vi "Newmark-Jog.vi"(0 "Table VRN IN":refnum<visa-resource-name>="COM9", 1 "StageTag":string, 2 "Bool Refnum":refnum<vi>, 11 "Error IN":errorcluster, 13 "Velocity":dbl) -> (4 "Table VRN OUT":refnum<visa-resource-name>="COM9", 15 "Error OUT":errorcluster)   [LabVIEW 2011]
uses:
  Comm/SerialCommError.vi
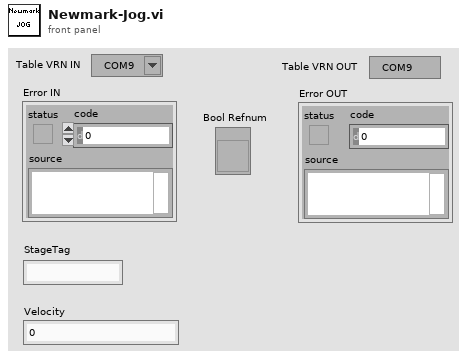
[diagram p1: front panel]
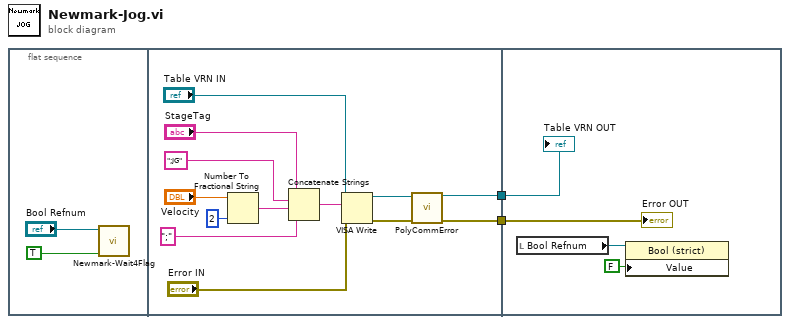
[diagram p0: block diagram]
diagram:
  n1 = flat-sequence {
    tunnel: [w15] -> w2
    tunnel: [w14] -> w1
    tunnel: w2 -> [w20]
    tunnel: w1 -> [w19]
    frame #0 {
      n2 = call "Newmark-Wait4Flag.vi"("Raise Flag ?"=TRUE, "Ctl Refnum IN"="Bool Refnum") -> ()  [unwired: 8 in, 2 out]
    }
    frame #1 {
      n3 = Number To Fractional String(number="Velocity", precision (6)=i16 2) -> (F-format string=w8:string)  [unwired: 2 in]
      n4 = Concatenate Strings("StageTag", ";JG", w8, ";") -> (w5:string)
      n5 = VISA Write(VISA resource name="Table VRN IN", write buffer=w5, error in (no error)="Error IN") -> (VISA resource name out=w17:refnum<visa-resource-name>, error out=w16:errorcluster)  [unwired: 1 out]
      n6 = call-poly "PolyCommError.vi"("VISA IN"=w17, "error IN"=w16) -> ("VISA OUT"=w15:refnum<visa-resource-name>, "error OUT"=w14:errorcluster)  [unwired: 11 in, 1 out]
    }
    frame #2 {
      n7 = local read "Bool Refnum"() -> (w18:refnum<vi>)
      n8 = property class="Bool (strict)"(reference=w18, "Value"=FALSE) -> ()  [unwired: 1 in, 2 out]
      "Table VRN OUT" <- w20
      "Error OUT" <- w19
    }
  }
